vi "power analyzer - Copy.vi"() -> ()   [LabVIEW 2011]
uses:
  <instrlib>/Voltech PM1000+/Voltech PM1000+.lvlib
panel:
  out "Measurement Results":string[][](array[string])
  in  "Set Start Time (s)":dbl
  in  "Time Target (s)":dbl=8.0
  out "stripped path":path
  out "error out":errorcluster
  in  "VISA resource name 2":refnum<visa-resource-name>
  in  "Team (eg. Instrumentation)":string
  in  "Name (First and Last)":string
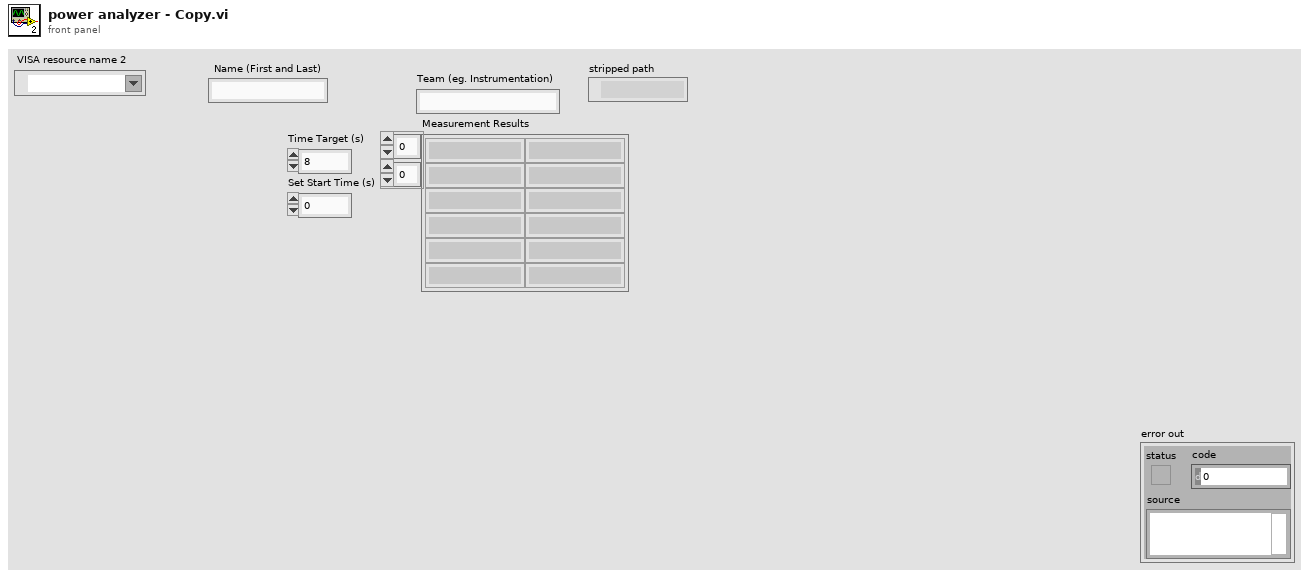
[diagram p1: front panel]
types:
  T1 = enum16{"open", "replace", "create", "open or create", "replace or create", "replace or create with confirmation"}
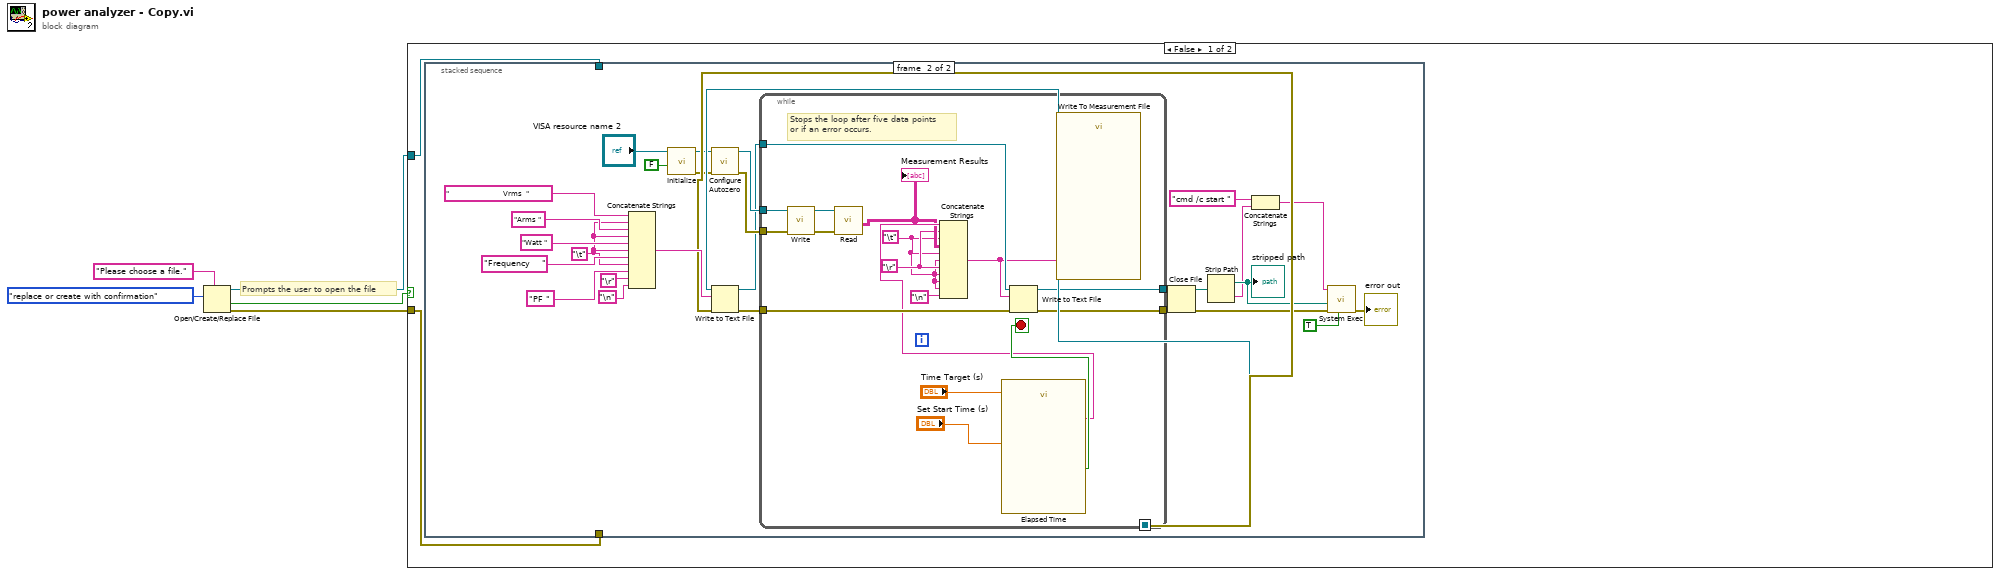
[diagram p0: block diagram]
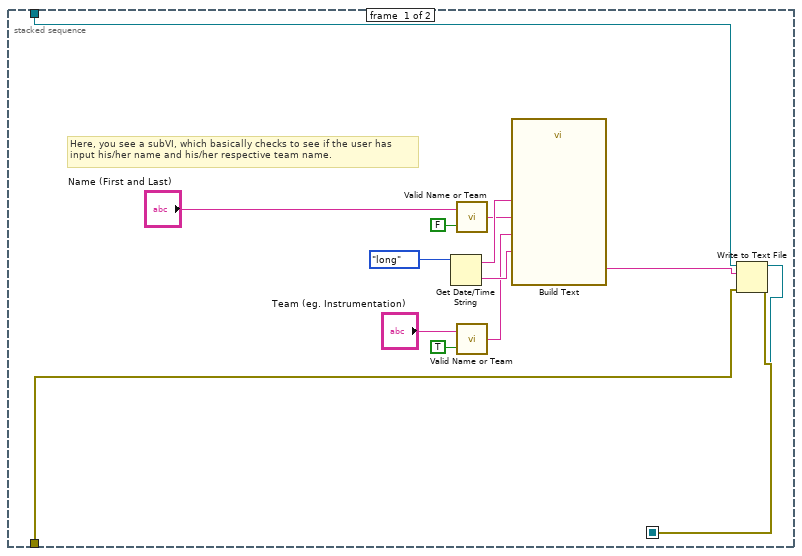
[diagram p2: hidden frame]
diagram:
  # "Prompts the user to open the file"
  n1 = Open/Create/Replace File(prompt="Please choose a file.", operation (0:open)=T1."replace or create with confirmation") -> (refnum out=w3:refnum<file>, cancelled=w1:bool, error out=w2:errorcluster)  [unwired: 4 in]
  n2 = case shown="False" w1 {
    tunnel: w3 -> [w6 _]
    tunnel: w2 -> [w7 _]
    frame False {
      n3 = stacked-sequence {
        seq-local: [w9 _] -> [_ w41]
        seq-local: [w8 _] -> [_ w40]
        tunnel: w7 -> [w11 _]
        tunnel: w6 -> [w10 _]
        frame #0 {
          # "Here, you see a subVI, which basically checks to see if the user has\ninput his/her name and his/her respective team name."
          n4 = Get Date/Time String(date format (0)=enum16{"short", "long", "abbreviated"}."long") -> (date string=w19:string, time string=w20:string)  [unwired: 2 in]
          n5 = call "Valid Name or Team.vi"("Input Boolean"=FALSE, "Input String"="Name (First and Last)") -> ("Output String"=w17:string)
          n6 = call "Valid Name or Team.vi"("Input Boolean"=TRUE, "Input String"="Team (eg. Instrumentation)") -> ("Output String"=w18:string)
          n7 = call "Build Text"("Time"=w20, "Name"=w17, "Team"=w18, "Date"=w19) -> ("Result"=w21:string)  [unwired: 10 in, 1 out]
          n8 = Write to Text File(file (use dialog)=w10, text=w21, error in=w11) -> (refnum out=w8:refnum<file>, error out=w9:errorcluster)  [unwired: 1 in, 1 out]
        }
        frame #1 {
          w45 = "\t"
          n9 = Concatenate Strings("                           Vrms  " ("string"), w45, "Arms " ("string"), w45, "Watt " ("string"), w45, "Frequency    " ("string"), w45, "PF " ("string"), "\r", "\n") -> (w47:string)
          n10 = call <instrlib>:"Initialize.vi"("Reset (True)"=FALSE, "VISA resource name"="VISA resource name 2") -> ("error out"=w37:errorcluster, "VISA resource name out"=w36:refnum<visa-resource-name>)  [unwired: 8 in]
          n11 = call <instrlib>:"Configure Autozero.vi"("error in (no error)"=w37, "VISA resource name"=w36) -> ("error out"=w33:errorcluster, "VISA resource name out"=w34:refnum<visa-resource-name>)  [unwired: 8 in]
          n12 = Write to Text File(file (use dialog)=w40, text=w47, error in=w41) -> (refnum out=w32:refnum<file>, error out=w39:errorcluster)  [unwired: 1 in, 1 out]
          n13 = while {
            tunnel: w39 -> [w67]
            tunnel: w34 -> [w60]
            tunnel: w33 -> [w59]
            tunnel: w32 -> [w64]
            tunnel: [w63] -> w23
            tunnel: [w62] -> w22
            stop <- w56 stop-if-true
            w52 = "\t"
            w53 = "\r"
            # "Stops the loop after five data points\nor if an error occurs."
            n14 = call <instrlib>:"Write.vi"("error in (no error)"=w59, "VISA resource name"=w60) -> ("error out"=w65:errorcluster, "VISA resource name out"=w66:refnum<visa-resource-name>)  [unwired: 8 in]
            n15 = call <instrlib>:"Read.vi"("error in (no error)"=w65, "VISA resource name"=w66) -> ("Measurement Results"=w54:string[][])  [unwired: 7 in, 2 out]
            "Measurement Results" <- w54
            n16 = call "Elapsed Time"("Time Target (s)"="Time Target (s)", "Set Start Time (s)"="Set Start Time (s)") -> ("Time has Elapsed"=w56:bool, "Elapsed Time Text"=w55:string)  [unwired: 10 in, 6 out]
            n17 = Concatenate Strings(w55, w53, w52, w54, w52, w52, w53, w52, w52, w52, "\n") -> (w51:string)
            n18 = Write to Text File(file (use dialog)=w64, text=w51, error in=w67) -> (refnum out=w62:refnum<file>, error out=w63:errorcluster)  [unwired: 1 in, 1 out]
            n19 = call "Write To Measurement File"("Comment"=w51) -> ()  [unwired: 16 in, 3 out]
          }
          n20 = Close File(refnum=w22, error in=w23) -> (path=w27:path, error out=w30:errorcluster)
          n21 = Strip Path(path=w27) -> (stripped path=w29:path, name=w28:string)
          "stripped path" <- w29
          n22 = Concatenate Strings("cmd /c start " ("string"), w28) -> (w26:string)
          n23 = call <vilib>:"System Exec.vi"("run minimized? (F)"=TRUE, "error in (no error)"=w30, "working directory"=w29, "command line"=w26) -> ("error out"=→"error out":errorcluster)  [unwired: 4 in, 3 out]
        }
      }
    }
    frame True {
    }
  }
